vi "main.vi"() -> ()   [LabVIEW 2020]
uses:
  <vilib>/JDP Science/JSONtext/Next JSON Value.vi
  <vilib>/JDP Science/JSONtext/String Subset.vi
  <vilib>/JDP Science/JSONtext/Parsing/Advance past next JSON Value (inlined COPY).vi
  <vilib>/JDP Science/JSONtext/Parsing/Advance past whitespace.vi
  <vilib>/JDP Science/JSONtext/Parsing/Advance past String.vi
  <vilib>/JDP Science/JSONtext/Parsing/Advance past Number.vi
  <vilib>/JDP Science/JSONtext/Parsing/Advance past Line Ending.vi
  <vilib>/JDP Science/JSONtext/Parsing/Parse Full Path or Item Name.vi
  <vilib>/JDP Science/JSONtext/Parsing/Advance past Array.vi
  <vilib>/JDP Science/JSONtext/Parsing/Advance past Object.vi
  <vilib>/JDP Science/JSONtext/support/Error Cluster From Code.vi
  <vilib>/JDP Science/JSONtext/Offset/Find Item Locations by Path.vi
  <vilib>/Utility/traverseref.llb/VI Scripting - Traverse.lvlib
  <vilib>/Utility/traverseref.llb/TRef TravTarget.ctl
  <vilib>/JDP Science/JSONtext/JSONtext.lvlib
panel:
  out "<JSON> 2":string caption="<JSON>Item"
  out "VI路径":path
  out "数组":string[](array[string])
  out "<JSON>":string
  in  "Path to Entrance VI":path=path "C:/Users/Fred/Desktop/LabAI/main.vi"
  # "C:\\Users\\Fred\\Desktop\\LabAI\\main.vi"
  # "C:\\Users\\Fred\\Desktop\\FL62风洞主控软件\\Desktop\\2.4米风洞主控软件20240716\\重排后重组.vi"
  # "C:\\Users\\Fred\\Desktop\\FL62风洞主控软件\\Desktop\\2.4米风洞主控软件20240716\\主程序 - 一键启动-web.vi"
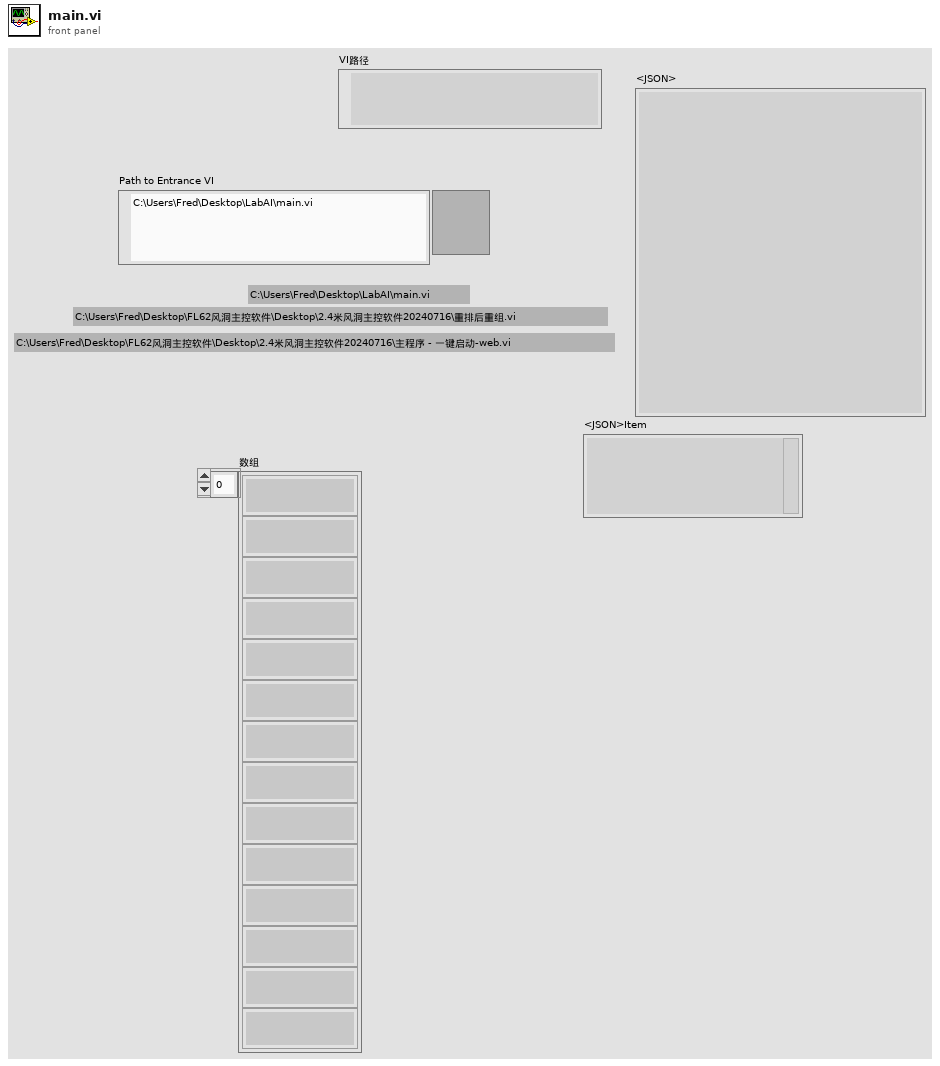
[diagram p1: front panel]
types:
  T1 = typedef "TRef TravTarget.ctl" = enum16{"FP", "BD", "Other"}
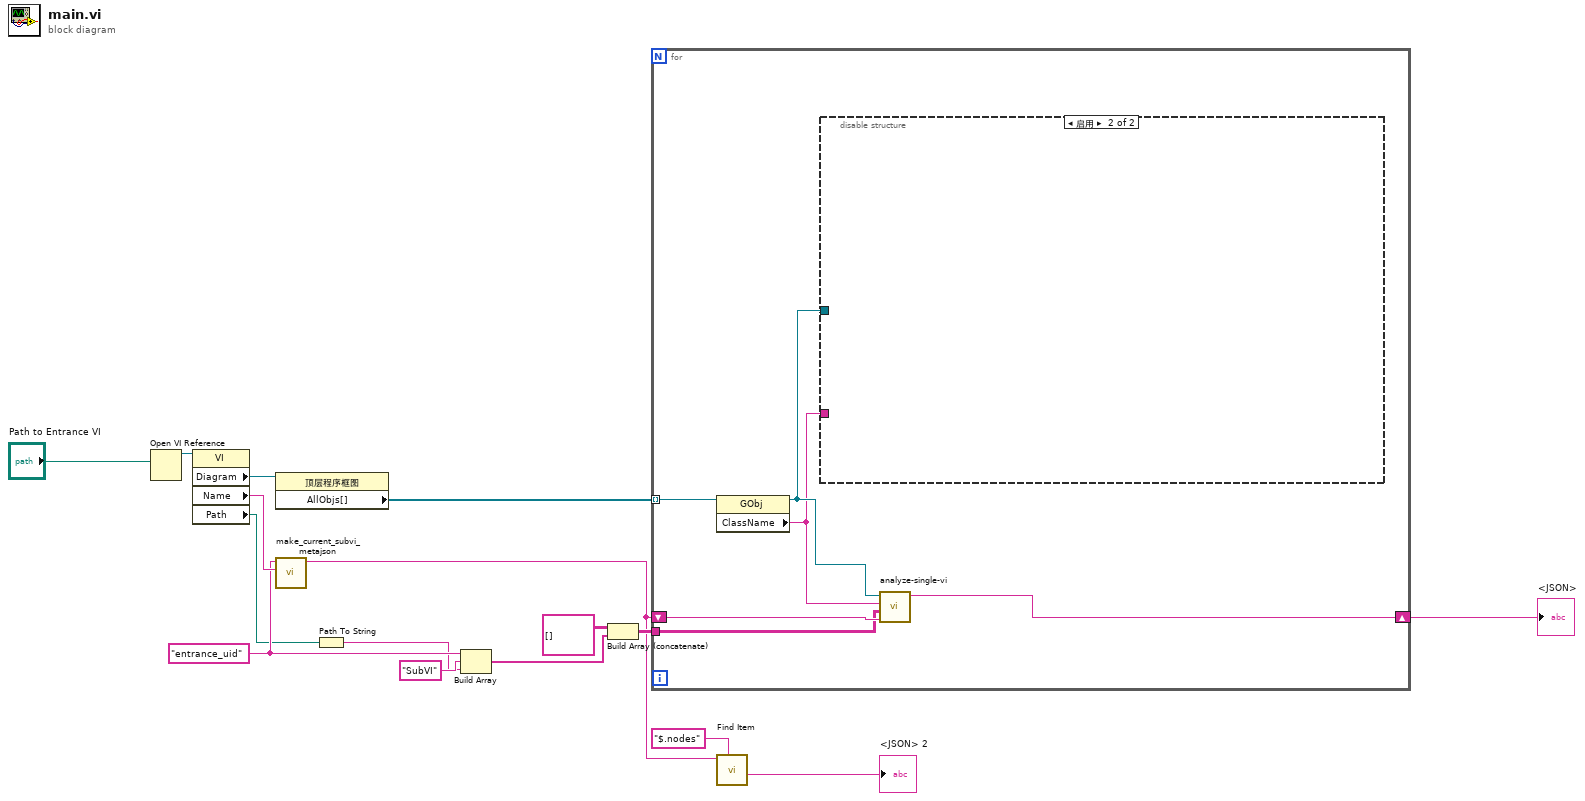
[diagram p0: block diagram]
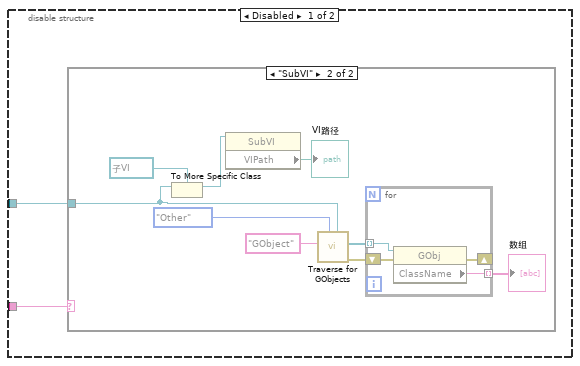
[diagram p2: hidden frame]
diagram:
  w10 = "entrance_uid" ("uid")
  n1 = Open VI Reference(vi path="Path to Entrance VI") -> (vi reference=w15:refnum<vi>)  [unwired: 5 in, 1 out]
  n2 = property class="VI"(reference=w15) -> ("Diagram"=w14:refnum<vi>, "Name"=w12:string, "Path"=w9:path)  [unwired: 1 in, 2 out]
  n3 = property class="顶层程序框图"(reference=w14) -> ("AllObjs[]"=w13:refnum<vi>[])  [unwired: 1 in, 2 out]
  n4 = call "make_current_subvi_metajson.vi"("VIName"=w12, "uid"=w10) -> ("<JSON>"=w3:string)  [unwired: 9 in]
  n5 = Path To String(path=w9) -> (string=w8:string)
  n6 = Build Array(w10, "SubVI" ("y"), w8) -> (w6:string[])
  n7 = Build Array (concatenate)(string[][] [] ("context"), w6) -> (w5:string[][])
  n8 = for {
    tunnel: w13 -> [w22] mode=indexing
    shift-right: [w20] -> w1
    shift-left: w3 -> [w21]
    tunnel: w5 -> [w19]
    n9 = property class="GObj"(reference=w22) -> (reference out=w18:refnum<vi>, "ClassName"=w17:string)  [unwired: 1 in, 1 out]
    n10 = disable-structure shown="启用" {
      disable-tunnel: w17 -> [w24 _]
      disable-tunnel: w18 -> [w23 _]
      frame Disabled {
        n11 = case shown="\"SubVI\"" w24 {
          tunnel: w23 -> [_ w27]
          frame "假", Default {
          }
          frame "SubVI" {
            n12 = To More Specific Class(target class=refnum<vi> refnum ("引用"), reference=w27) -> (specific class reference=w26:refnum<vi>)  [unwired: 1 in, 1 out]
            n13 = property class="SubVI"(reference=w26) -> ("VIPath"=→"VI路径":path)  [unwired: 1 in, 2 out]
            n14 = call <vilib>:"Traverse for GObjects.vi"("Other Refnum"=w27, "Traverse Target"=TRef_TravTarget."Other", "Class Name"="GObject") -> ("error out"=w31:errorcluster, "References"=w30:refnum<vi>[])  [unwired: 5 in, 2 out]
            n15 = for {
              tunnel: w30 -> [w37] mode=indexing
              tunnel: [w36] -> w29 mode=indexing
              shift-right: [w34] -> _
              shift-left: w31 -> [w35]
              n16 = property class="GObj"(reference=w37, error in=w35) -> (error out=w34:errorcluster, "ClassName"=w36:string)  [unwired: 1 out]
            }
            "数组" <- w29
          }
        }
      }
      frame Enabled {
      }
    }
    n17 = call "analyze-single-vi.vi"("GObj引用句柄"=w18, "type"=w17, "context"=w19, "json_input"=w21) -> ("<JSON> 3"=w20:string)  [unwired: 6 in]
  }
  "<JSON>" <- w1
  n18 = call <vilib>:"Find Item.vi"("$Path or Item Name"="$.nodes", "JSON"=w3) -> ("<JSON>"=→"<JSON> 2":string)  [unwired: 6 in, 3 out]
